vi "lv create stream.vi"(8 "error in":errorcluster, 10 "dataset handle":i32, 11 "client handle":i32) -> (0 "error out":errorcluster, 3 "stream handle":i32)   [LabVIEW 2026]
uses:
  bin/nominalClient_64.dll
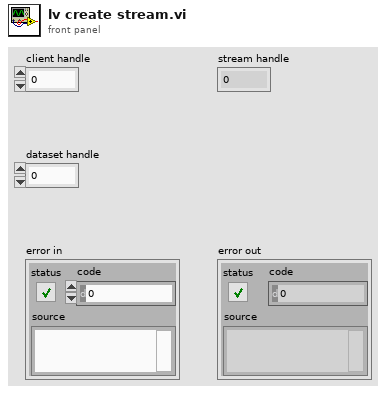
[diagram p1: front panel]
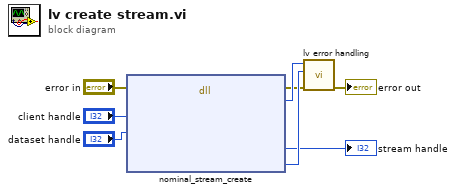
[diagram p0: block diagram]
diagram:
  n1 = dll-call lib="C:/sw/nominal-c/bin/nominalClient_64.dll" fn="nominal_stream_create"(error in="error in", "client"="client handle", "dataset handle"="dataset handle") -> (error out=w5:errorcluster, "return type"=w7:i32, "stream handle"=→"stream handle":i32, "errorout"=w8:i32)  [unwired: 6 in, 1 out]
  n2 = call "lv error handling.vi"("error in"=w5, "error handle"=w8, "return code"=w7) -> ("error out"=→"error out":errorcluster)  [unwired: 8 in]
